vi "Hypergeometric Inverse CDF.vi"(8 "n":i32=20, 9 "k":i32=30, 10 "M":i32=100, 11 "cdf(x)":dbl=0.209163) -> (0 "error":i32, 3 "x":i32=4)   [LabVIEW 2020, in "NI_Gmath.lvlib"]
doc: "Computes the discrete inverse cumulative distribution function (CDF), or the value <B>x</B> such that the probability that the random variate X, where X describes the selected distribution type, takes on a value less than or equal to it is <B>cdf(x)</B>. You must manually select the polymorphic instance to use."
uses:
  NI_Gmath.lvlib
panel:
  # "Hypergeometric Inverse CDF"
  # "size of population"
  # "items"
  # "samples drawn"
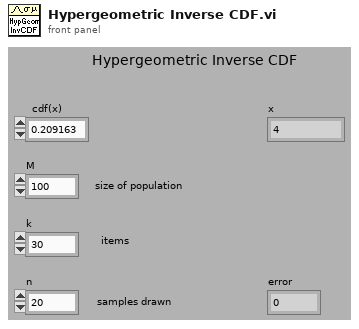
[diagram p1: front panel]
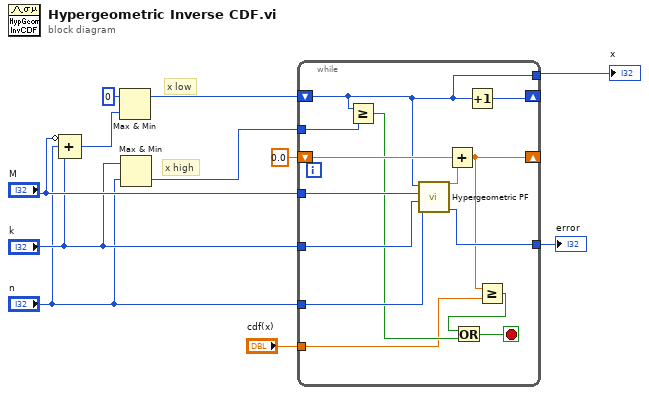
[diagram p0: block diagram]
diagram:
  # "x high"
  # "x low"
  n1 = Compound Arithmetic op=ADD(invert "M", "n", "k") -> (w7:i32)
  n2 = Max & Min(x=0, y=w7) -> (max(x,y)=w4:i32)  [unwired: 1 out]
  n3 = Max & Min(x="k", y="n") -> (min(x,y)=w3:i32)  [unwired: 1 out]
  n4 = while {
    tunnel: [w25] -> w11
    tunnel: "M" -> [w24]
    tunnel: "k" -> [w23]
    tunnel: "n" -> [w22]
    shift-right: [w17] -> _
    shift-left: 0.0 -> [w20]
    shift-right: [w19] -> _
    shift-left: w4 -> [w12]
    tunnel: w3 -> [w18]
    tunnel: "cdf(x)" -> [w14]
    tunnel: [w12] -> w1
    stop <- w13 stop-if-true
    n5 = Greater Or Equal?(x=w12, y=w18) -> (x >= y?=w16:bool)
    n6 = call "Hypergeometric PF.vi"("n"=w22, "k"=w23, "M"=w24, "x"=w12) -> ("error"=w25:i32, "prob(x)"=w21:dbl)  [unwired: 6 in]
    n7 = Add(x=w20, y=w21) -> (x+y=w17:dbl)
    n8 = Increment(x=w12) -> (x+1=w19:i32)
    n9 = Greater Or Equal?(x=w17, y=w14) -> (x >= y?=w15:bool)
    n10 = Or(x=w15, y=w16) -> (x .or. y?=w13:bool)
  }
  "x" <- w1
  "error" <- w11
